vi "String Array Remove Duplicate Typedefinitions.vi"(1 "Array":string[](array[string])) -> (0 "Output array":string[](array[string]))   [LabVIEW 2014]
doc: "Delete duplicate items in String array."
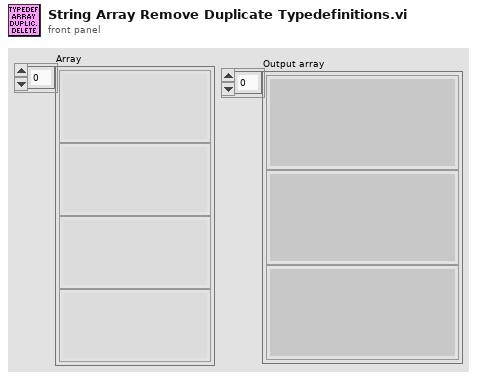
[diagram p1: front panel]
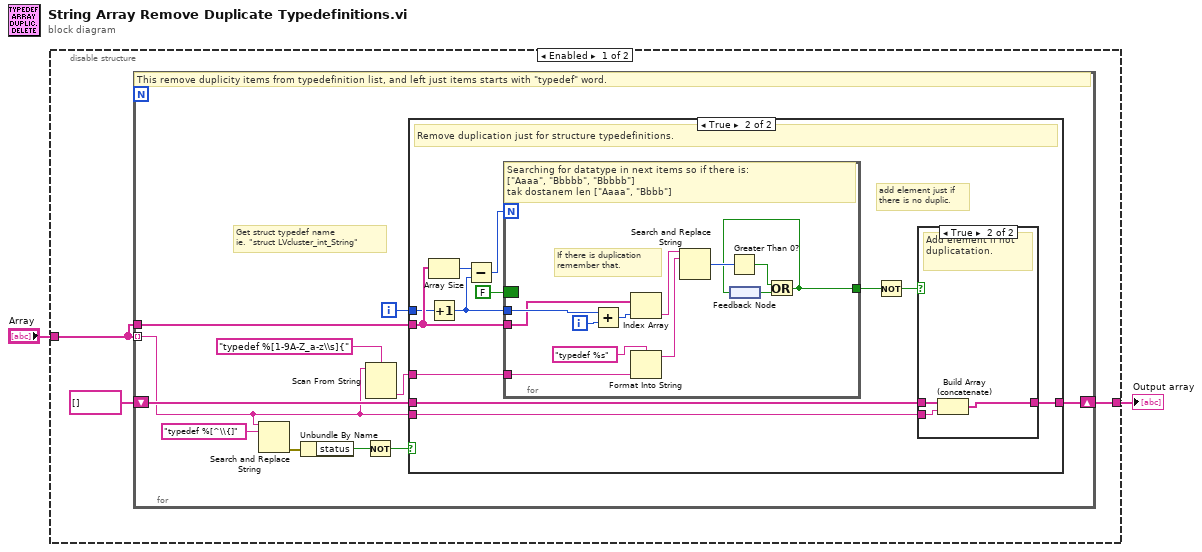
[diagram p0: block diagram]
diagram:
  n1 = disable-structure shown="Enabled" {
    disable-tunnel: [w5 w46] -> w2
    disable-tunnel: "Array" -> [w3 w46]
    frame Enabled {
      n2 = for {
        shift-right: [w16] -> w5
        shift-left: string[] [] -> [w15]
        tunnel: w3 -> [w6] mode=indexing
        tunnel: w3 -> [w14]
        i -> [w13]
        # "Get struct typedef name\nie. \"struct LVcluster_int_String\""
        # "This remove duplicity items from typedefinition list, and left just items starts with \"typedef\" word."
        n3 = Search and Replace String(input string=w6, search string="typedef %[^\\{]" ("format string")) -> (error out=w9:errorcluster)  [unwired: 6 in, 3 out]
        n4 = Unbundle By Name(w9) -> ("status"=w12:bool)
        n5 = Not(x=w12) -> (.not. x?=w11:bool)
        n6 = Scan From String(format string="typedef %[1-9A-Z_a-z\\s]{", input string=w6) -> (output 1=w7:string)  [unwired: 3 in, 3 out]
        n7 = case shown="True" w11 {
          tunnel: w7 -> [_ w23]
          tunnel: [w17 w25] -> w16
          tunnel: w15 -> [w17 w24]
          tunnel: w14 -> [_ w28]
          tunnel: w13 -> [_ w26]
          tunnel: w6 -> [_ w18]
          frame False {
          }
          frame True {
            # "add element just if\nthere is no duplic."
            # "Remove duplication just for structure typedefinitions."
            n8 = Array Size(array=w28) -> (size(s)=w29:i32)
            n9 = Increment(x=w26) -> (x+1=w19:i32)
            n10 = Subtract(x=w29, y=w19) -> (x-y=w27:i32)
            n11 = for {
              N: w27 -> [_]
              tunnel: w28 -> [w40]
              tunnel: w19 -> [w43]
              tunnel: w23 -> [w41]
              tunnel: [w34] -> w21
              border: FALSE -> [_]
              i -> [w45]
              # "If there is duplication remember that."
              # "Searching for datatype in next items so if there is:\n[\"Aaaa\", \"Bbbbb\", \"Bbbbb\"]\ntak dostanem len [\"Aaaa\", \"Bbbb\"]"
              n12 = Add(x=w43, y=w45) -> (x+y=w44:i32)
              n13 = Index Array(array=w40, index=w44) -> (element=w38:string)
              n14 = Format Into String(format string="typedef %s", w41) -> (resulting string=w39:string)  [unwired: 2 in, 1 out]
              n15 = Search and Replace String(input string=w38, search string=w39) -> (number of replacements=w37:i32)  [unwired: 6 in, 3 out]
              n16 = Greater Than 0?(x=w37) -> (x > 0?=w36:bool)
              n17 = feedback #1() -> (w35:bool)
              n18 = Or(x=w36, y=w35) -> (x .or. y?=w34:bool)
              n19 = feedback-in #1(w34) -> ()
            }
            n20 = Not(x=w21) -> (.not. x?=w22:bool)
            n21 = case shown="True" w22 {
              tunnel: [w30 w33] -> w25
              tunnel: w24 -> [w30 w32]
              tunnel: w18 -> [_ w31]
              frame False {
              }
              frame True {
                # "Add element if not duplicatation."
                n22 = Build Array (concatenate)(w32, w31) -> (w33:string[])
              }
            }
          }
        }
      }
    }
    frame Disabled {
    }
  }
  "Output array" <- w2
